vi "3_Wheels_Facade.vi"(0 "Data In":T4={"InCluster"={"MotorSpeed0"=0.0, "MotorSpeed1"=0.0, "MotorSpeed2"=0.0, "MotorSpeed3"=0.0, "HCDIO 1"=0.0, "HCDIO 2"=0.0, "HCDIO 3"=0.0, "HCDIO 4"=0.0, "HCDIO 5"=0.0, "HCDIO 6"=0.0, "HCDIO 7"=0.0, "HCDIO 8"=0.0, "HCDIO 9"=0.0, "HCDIO 10"=0.0}, "In_Cluster"={"MotorEnc0"=0.0, "MotorEnc1"=0.0, "MotorEnc2"=0.0, "MotorEnc3"=0.0, "US1"=0.0, "US2"=0.0, "Analog1"=0.0, "Analog2"=0.0, "Analog3"=0.0, "Analog4"=0.0, "IMU"=0.0, "TitanLimits"=[FALSE, FALSE, FALSE, FALSE, FALSE, FALSE, FALSE, FALSE], "Flexs"=[FALSE, FALSE, FALSE, FALSE, FALSE, FALSE, FALSE, FALSE], "Camera"="RobocadImage"}}, 2 "Display State In":T2, 3 "Container State":T3) -> (6 "Data Out":T4={"InCluster"={"MotorSpeed0"=0.0, "MotorSpeed1"=0.0, "MotorSpeed2"=0.0, "MotorSpeed3"=0.0, "HCDIO 1"=0.0, "HCDIO 2"=0.0, "HCDIO 3"=0.0, "HCDIO 4"=0.0, "HCDIO 5"=0.0, "HCDIO 6"=0.0, "HCDIO 7"=0.0, "HCDIO 8"=0.0, "HCDIO 9"=0.0, "HCDIO 10"=0.0}, "In_Cluster"={"MotorEnc0"=0.0, "MotorEnc1"=0.0, "MotorEnc2"=0.0, "MotorEnc3"=0.0, "US1"=0.0, "US2"=0.0, "Analog1"=0.0, "Analog2"=0.0, "Analog3"=0.0, "Analog4"=0.0, "IMU"=0.0, "TitanLimits"=[FALSE, FALSE, FALSE, FALSE, FALSE, FALSE, FALSE, FALSE], "Flexs"=[FALSE, FALSE, FALSE, FALSE, FALSE, FALSE, FALSE, FALSE], "Camera"="RobocadImage"}}, 7 "Display State Out":T2, 8 "Action":T1)   [LabVIEW 2019, in "3_Wheels.xctl"]
uses:
  3_Wheels.xctl
  3_Wheels.ctl
  <vilib>/vision/Image Controls.llb/IMAQ Image.ctl
  <vilib>/_xctls/Container State.ctl
  3_Wheels_Robot.ctl
  <vilib>/_xctls/Action.ctl
  <vilib>/_xctls/XControlSupport.lvlib
panel:
  out "Enc_2":dbl
  out "Enc_1":dbl
  out "Enc_0":dbl
  out "Motor_2":dbl
  out "Motor_1":dbl
  out "Motor_0":dbl
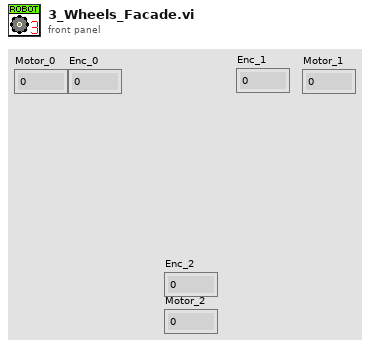
[diagram p1: front panel]
types:
  T1 = typedef "XControlSupport.lvlib/Action.ctl" = cluster{"Data Changed?":bool, "State Changed?":bool, "Action Name":string}
  T2 = typedef "3_Wheels.xctl/3_Wheels_Robot.ctl" = cluster{"Numeric":dbl}
  T3 = typedef "XControlSupport.lvlib/Container State.ctl" = cluster{"Indicator?":bool, "Run Mode?":bool, " Refnum":refnum<vi>}
  T4 = typedef "3_Wheels.xctl/3_Wheels.ctl" = cluster{"InCluster":cluster{"MotorSpeed0":dbl, "MotorSpeed1":dbl, "MotorSpeed2":dbl, "MotorSpeed3":dbl, "HCDIO 1":dbl, "HCDIO 2":dbl, "HCDIO 3":dbl, "HCDIO 4":dbl, "HCDIO 5":dbl, "HCDIO 6":dbl, "HCDIO 7":dbl, "HCDIO 8":dbl, "HCDIO 9":dbl, "HCDIO 10":dbl}, "In_Cluster":cluster{"MotorEnc0":dbl, "MotorEnc1":dbl, "MotorEnc2":dbl, "MotorEnc3":dbl, "US1":dbl, "US2":dbl, "Analog1":dbl, "Analog2":dbl, "Analog3":dbl, "Analog4":dbl, "IMU":dbl, "TitanLimits":bool[], "Flexs":bool[], "Camera":T5}}
  T5 = typedef "IMAQ Image.ctl" = refnum<image>
  T6 = cluster{"MotorSpeed0":dbl, "MotorSpeed1":dbl, "MotorSpeed2":dbl, "MotorSpeed3":dbl, "HCDIO 1":dbl, "HCDIO 2":dbl, "HCDIO 3":dbl, "HCDIO 4":dbl, "HCDIO 5":dbl, "HCDIO 6":dbl, "HCDIO 7":dbl, "HCDIO 8":dbl, "HCDIO 9":dbl, "HCDIO 10":dbl}
  T7 = cluster{"MotorEnc0":dbl, "MotorEnc1":dbl, "MotorEnc2":dbl, "MotorEnc3":dbl, "US1":dbl, "US2":dbl, "Analog1":dbl, "Analog2":dbl, "Analog3":dbl, "Analog4":dbl, "IMU":dbl, "TitanLimits":bool[], "Flexs":bool[], "Camera":T5}
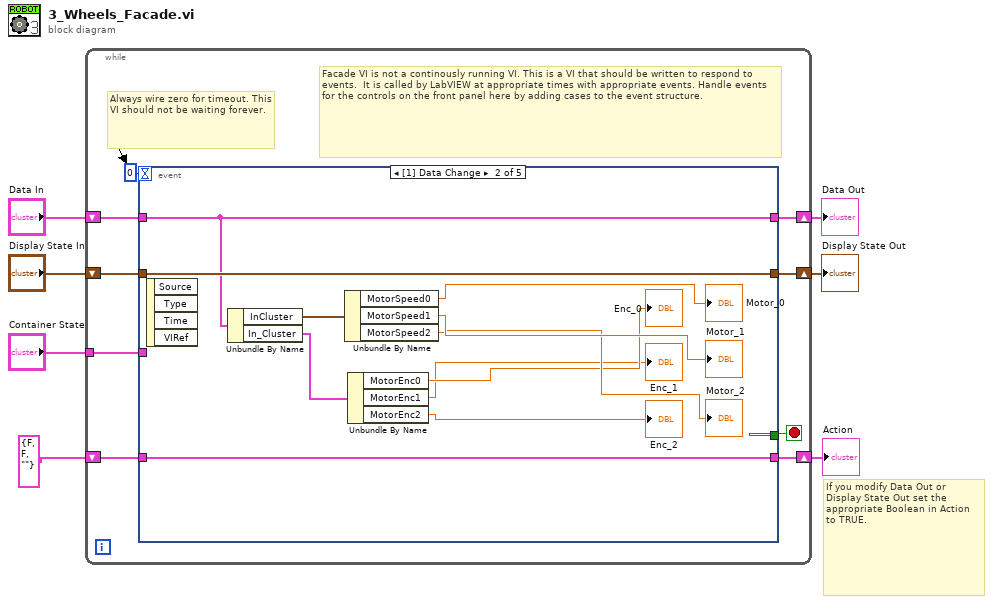
[diagram p0: block diagram]
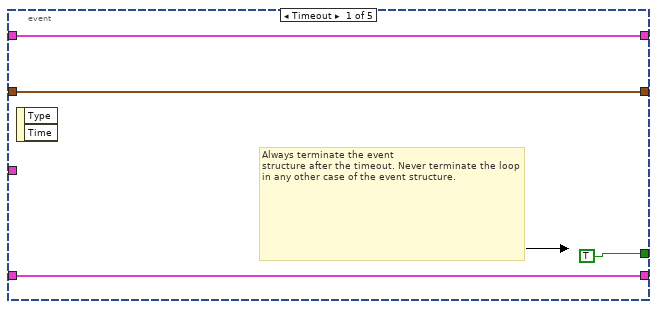
[diagram p2: hidden frame]
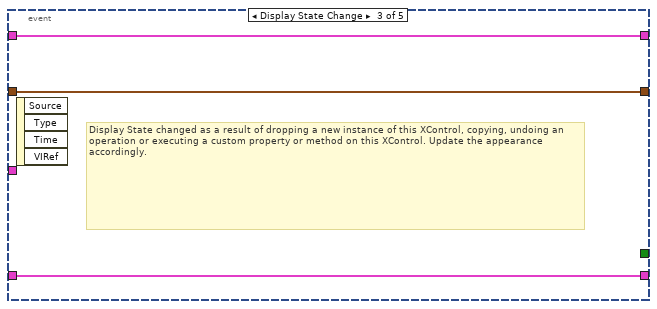
[diagram p3: hidden frame]
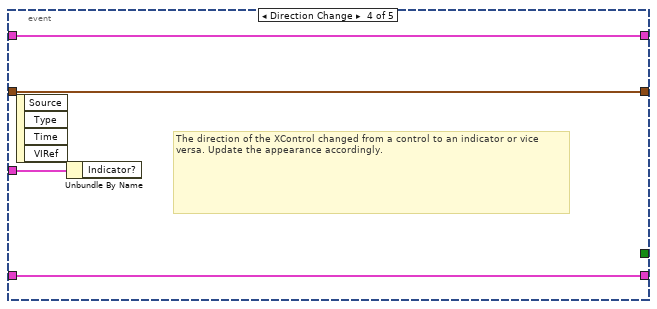
[diagram p4: hidden frame]
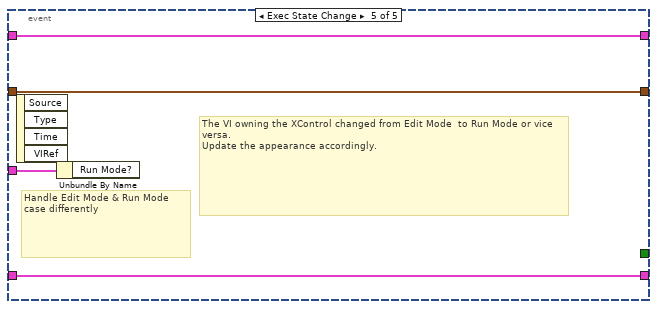
[diagram p5: hidden frame]
diagram:
  # "If you modify Data Out or\nDisplay State Out set the\nappropriate Boolean in Action\nto TRUE."
  n1 = while {
    shift-right: [w15] -> w4
    shift-left: "Display State In" -> [w16]
    tunnel: "Container State" -> [w12]
    shift-right: [w10] -> w7
    shift-left: "Data In" -> [w11]
    shift-right: [w8] -> w2
    shift-left: T1 {"Data Changed?"=FALSE, "State Changed?"=FALSE, "Action Name"=""} ("Action") -> [w9]
    stop <- w14 stop-if-true
    # "Facade VI is not a continously running VI. This is a VI that should be written to respond to events.  It is called by LabVIEW at appropriate times with appropriate events. Handle events for the controls on the front panel here by adding cases to the event structure."
    # "Always wire zero for timeout. This\nVI should not be waiting forever."
    n2 = event shown="[1] Data Change" {
      selector: _ -> [_ _ _ _ _]
      dyn-events: _ -> [_ _ _ _ _]
      timeout: 0 -> [_ _ _ _ _]
      tunnel: w16 -> [w18 w31 w34 w37 w41]
      tunnel: [w18 w31 w34 w37 w41] -> w15
      tunnel: [TRUE _ _ _ _] -> w14
      tunnel: w12 -> [_ _ _ w38 w42]
      tunnel: w11 -> [w17 w29 w33 w36 w40]
      tunnel: [w17 w29 w33 w36 w40] -> w10
      tunnel: [w19 w30 w32 w35 w39] -> w8
      tunnel: w9 -> [w19 w30 w32 w35 w39]
      event Timeout {
        # "Always terminate the event\nstructure after the timeout. Never terminate the loop in any other case of the event structure."
        n3 = event-data() -> ()  [unwired: 1 in, 2 out]
      }
      event Data Change {
        n4 = event-data() -> ()  [unwired: 1 in, 4 out]
        n5 = Unbundle By Name(w29) -> ("InCluster"=w28:T6, "In_Cluster"=w27:T7)
        n6 = Unbundle By Name(w28) -> ("MotorSpeed0"=→"Motor_0":dbl, "MotorSpeed1"=→"Motor_1":dbl, "MotorSpeed2"=→"Motor_2":dbl)
        n7 = Unbundle By Name(w27) -> ("MotorEnc0"=→"Enc_0":dbl, "MotorEnc1"=→"Enc_1":dbl, "MotorEnc2"=→"Enc_2":dbl)
      }
      event Display State Change {
        # "Display State changed as a result of dropping a new instance of this XControl, copying, undoing an operation or executing a custom property or method on this XControl. Update the appearance accordingly."
        n8 = event-data() -> ()  [unwired: 1 in, 4 out]
      }
      event Direction Change {
        # "The direction of the XControl changed from a control to an indicator or vice versa. Update the appearance accordingly."
        n9 = event-data() -> ()  [unwired: 1 in, 4 out]
        n10 = Unbundle By Name(w38) -> ()  [unwired: 1 out]
      }
      event Exec State Change {
        # "The VI owning the XControl changed from Edit Mode  to Run Mode or vice versa.\nUpdate the appearance accordingly."
        # "Handle Edit Mode & Run Mode\ncase differently"
        n11 = event-data() -> ()  [unwired: 1 in, 4 out]
        n12 = Unbundle By Name(w42) -> ()  [unwired: 1 out]
      }
    }
  }
  "Display State Out" <- w4
  "Data Out" <- w7
  "Action" <- w2
